vi "IQ to FXP18.vi"(2 "data in":T1[](array[typedef])=[{"I"=0.0, "Q"=0.0, "overflow"=FALSE}, {"I"=0.0, "Q"=0.0, "overflow"=FALSE}, {"I"=0.0, "Q"=0.0, "overflow"=FALSE}, {"I"=0.0, "Q"=0.0, "overflow"=FALSE}]) -> (7 "I out":fxp<+/-,18,1>[](array[numeric]), 9 "Q out":fxp<+/-,18,1>[](array[numeric]))   [LabVIEW 2018, in "GettingStarted_5774_FPGA.lvlib"]
uses:
  GettingStarted_5774_FPGA.lvlib
  <instrlib>/_niInstr/DSP/v1/Shared/Public/IQ Data.ctl
  <instrlib>/_niInstr/DSP/v1/Shared/niInstr DSP v1 Shared.lvlib
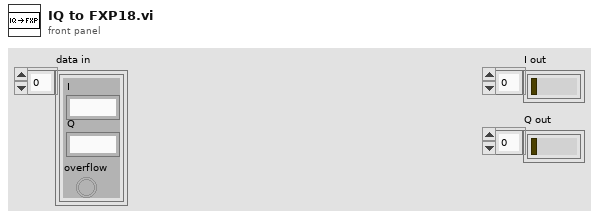
[diagram p1: front panel]
types:
  T1 = typedef "niInstr DSP v1 Shared.lvlib/IQ Data.ctl" = cluster{"I":fxp<+/-,18,1>, "Q":fxp<+/-,18,1>, "overflow":bool}
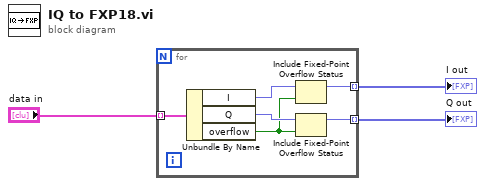
[diagram p0: block diagram]
diagram:
  n1 = for {
    tunnel: "data in" -> [w9] mode=indexing
    tunnel: [w5] -> w2 mode=indexing
    tunnel: [w4] -> w1 mode=indexing
    n2 = Unbundle By Name(w9) -> ("I"=w8:fxp<+/-,18,1>, "Q"=w7:fxp<+/-,18,1>, "overflow"=w6:bool)
    n3 = Include Fixed-Point Overflow Status(2:w6, 3:w8) -> (1:w5:fxp<+/-,18,1>)
    n4 = Include Fixed-Point Overflow Status(2:w6, 3:w7) -> (1:w4:fxp<+/-,18,1>)
  }
  "I out" <- w2
  "Q out" <- w1
